vi "TDT-Combine Channels and Codes.vi"(6 "offset":i32, 8 "Tetrode":bool, 9 "Times":dbl[](array[numeric]), 10 "Sort Codes":dbl[](array[numeric]), 11 "Channels":dbl[](array[numeric])) -> (1 "Times Out":dbl[](array[numeric]), 3 "Impale channel":dbl[](array[numeric]))   [LabVIEW 2020]
doc: "Converts TDT channel number and sort code pairs into a single Impale channel ID. Incorporating a sort code into Impale will break too many things, so we must send it scalar IDs. The unsorted spikes come in with a sort code of 31; we coerce that to MaxClusters + 1. MaxClusters defaults to the TDT-specified value of 5."
uses:
  <vilib>/Analysis/NI_AALPro.lvlib
panel:
  in  "Max Clusters":i32=5
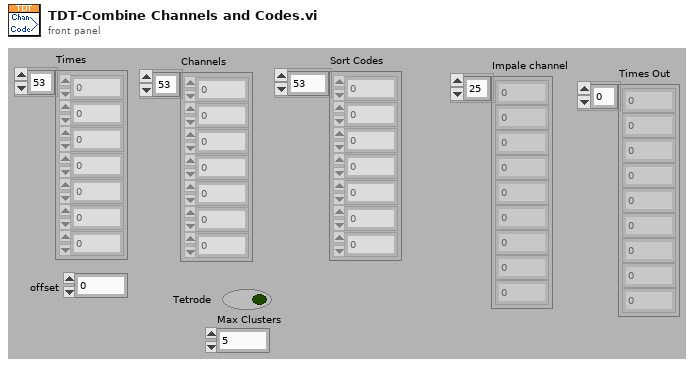
[diagram p1: front panel]
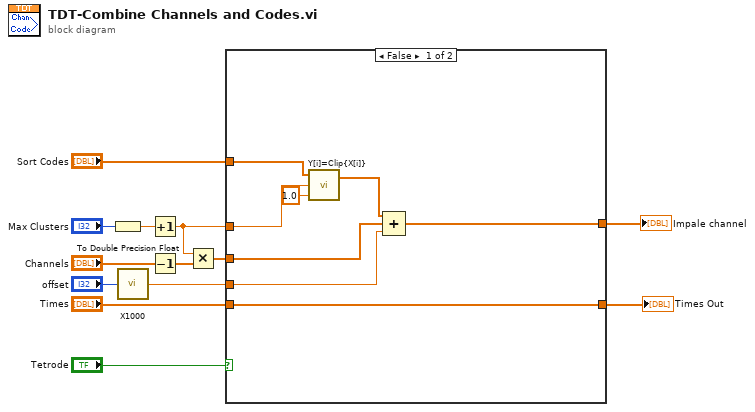
[diagram p0: block diagram]
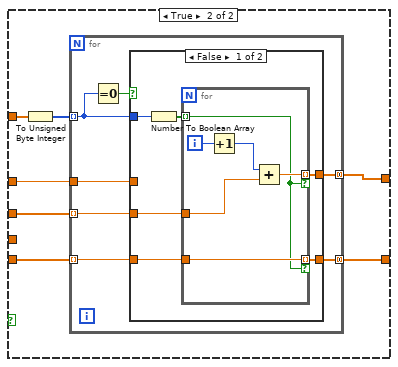
[diagram p2: hidden frame]
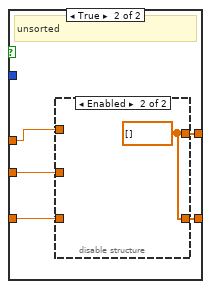
[diagram p3: hidden frame]
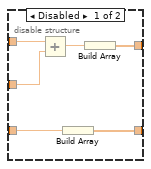
[diagram p4: hidden frame]
diagram:
  n1 = To Double Precision Float(number="Max Clusters") -> (double precision float=w3:dbl)
  n2 = call "X1000.vi"("X"="offset") -> ("X/1000"=w1:dbl)
  n3 = Increment(x=w3) -> (x+1=w7:dbl)
  n4 = Decrement(x="Channels") -> (x-1=w9:dbl[])
  n5 = Multiply(x=w7, y=w9) -> (x*y=w8:dbl[])
  n6 = case shown="False" "Tetrode" {
    tunnel: "Sort Codes" -> [w21 w28]
    tunnel: [w20 w25] -> w11
    tunnel: w8 -> [w17 w22]
    tunnel: w7 -> [w16 w26]
    tunnel: "Times" -> [w15 w27]
    tunnel: [w15 w24] -> w4
    tunnel: w1 -> [w14 _]
    frame False {
      n7 = call <vilib>:"Y[i]=Clip{X[i]}.vi"("lower limit"=1.0, "upper limit"=w16, "Input Array"=w21) -> ("Clipped Array"=w18:dbl[])  [unwired: 1 out]
      n8 = Compound Arithmetic op=ADD(w18, w17, w14) -> (w20:dbl[])
    }
    frame True {
      n9 = To Unsigned Byte Integer(number=w28) -> (unsigned 8bit integer=w23:u8[])
      n10 = for {
        tunnel: w23 -> [w30] mode=indexing
        tunnel: w27 -> [w33] mode=indexing
        tunnel: w26 -> [w34]
        tunnel: [w32] -> w25 mode=concatenating
        tunnel: [w31] -> w24 mode=concatenating
        tunnel: w22 -> [w29] mode=indexing
        n11 = Equal To 0?(x=w30) -> (x = 0?=w35:bool)
        n12 = case shown="False" w35 {
          tunnel: w34 -> [_ w52]
          tunnel: w33 -> [w40 w51]
          tunnel: [w37 w49] -> w32
          tunnel: [w36 w48] -> w31
          tunnel: w30 -> [w41 _]
          tunnel: w29 -> [w38 w50]
          frame False {
            n13 = Number To Boolean Array(number=w41) -> (Boolean array=w39:bool[])
            n14 = for {
              tunnel: w40 -> [w43]
              tunnel: w39 -> [w42] mode=indexing
              tunnel: w38 -> [w45]
              tunnel: [w44] -> w37 mode=indexing if=w42
              tunnel: [w43] -> w36 mode=indexing if=w42
              i -> [w47]
              n15 = Increment(x=w47) -> (x+1=w46:i32)
              n16 = Add(x=w46, y=w45) -> (x+y=w44:dbl)
            }
          }
          frame True {
            # "unsorted"
            n17 = disable-structure shown="Enabled" {
              disable-tunnel: w52 -> [w58 _]
              disable-tunnel: w51 -> [w57 _]
              disable-tunnel: w50 -> [w55 _]
              disable-tunnel: [w54 w59] -> w49
              disable-tunnel: [w53 w59] -> w48
              frame Disabled {
                n18 = Add(x=w58, y=w55) -> (x+y=w56:dbl)
                n19 = Build Array(w57) -> (w53:dbl[])
                n20 = Build Array(w56) -> (w54:dbl[])
              }
              frame Enabled {
                w59 = dbl[] []
              }
            }
          }
        }
      }
    }
  }
  "Impale channel" <- w11
  "Times Out" <- w4
